vi "Word to double.vi"(5 "ScaleOffset (0)":dbl, 7 "ScaleFac (1)":dbl=1.0, 8 "word":u32, 9 "Signed? (F)":bool, 10 "Number of Bits":T2=1 min=1 max=32, 11 "Start Bit":T1) -> (3 "Double":dbl)   [LabVIEW 2012, in "ARINC 429 Shared.lvlib"]
uses:
  Controls and Global/Number of Bits.ctl
  Controls and Global/Start Bit.ctl
  ARINC 429 Shared.lvlib
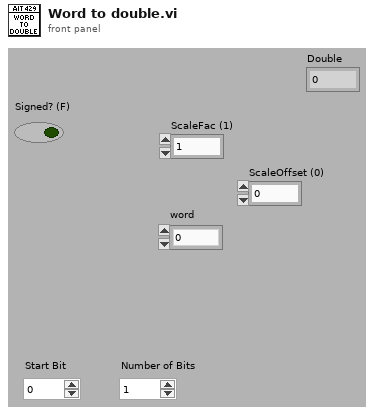
[diagram p1: front panel]
types:
  T1 = typedef "ARINC 429 Shared.lvlib/Start Bit.ctl" = i32
  T2 = typedef "ARINC 429 Shared.lvlib/Number of Bits.ctl" = i32
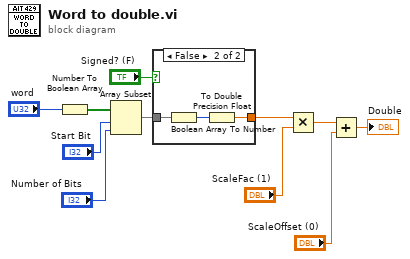
[diagram p0: block diagram]
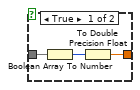
[diagram p2: hidden frame]
diagram:
  n1 = Number To Boolean Array(number="word") -> (Boolean array=w10:bool[])
  n2 = Array Subset(array=w10, index="Start Bit", length="Number of Bits") -> (w7:bool[])
  n3 = case shown="False" "Signed? (F)" {
    tunnel: w7 -> [w14 w17]
    tunnel: [w12 w15] -> w5
    frame True {
      n4 = Boolean Array To Number(Boolean array=w14) -> (number=w13:i32)
      n5 = To Double Precision Float(number=w13) -> (double precision float=w12:dbl)
    }
    frame False {
      n6 = Boolean Array To Number(Boolean array=w17) -> (number=w16:u32)
      n7 = To Double Precision Float(number=w16) -> (double precision float=w15:dbl)
    }
  }
  n8 = Multiply(x=w5, y="ScaleFac (1)") -> (x*y=w3:dbl)
  n9 = Add(x=w3, y="ScaleOffset (0)") -> (x+y=→"Double":dbl)
